vi "AddLifetimeData.vi"(0 "lower time (ms)":dbl, 1 "upper time (ms)":dbl, 2 "Decay":u32[][](array[numeric]), 3 "RAW data":T1) -> (8 "Decay out":u32[][](array[numeric]))   [LabVIEW 2009]
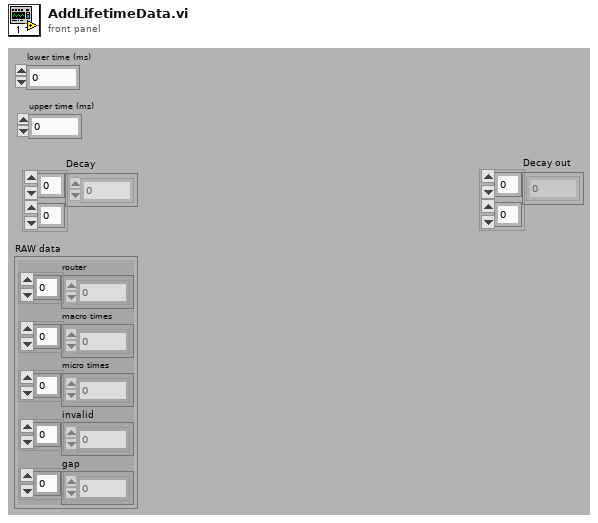
[diagram p1: front panel]
types:
  T1 = cluster{"router":u8[], "macro times":dbl[], "micro times":u16[], "invalid":dbl[], "gap":dbl[]}
  T2 = typedef "Settings.ctl" = cluster{"threshold":cluster{"max":u32, "min":u32}, "RGB or false color":bool, "16bit":bool, "log/lin axis":u16, "spotsize button":bool, "Pixelsize":u16, "autoscale x":bool, "autoscale y":bool, "correlation":bool, "ADC-Resolution":i32, "F2-lifetime":cluster{"display tau":bool, "display F2":bool, "Palette Number lifetime":enum32{"Gray", "Binary", "Gradient", "Rainbow", "Temperature"}, "Palette Number F2":enum32{"Gray", "Binary", "Gradient", "Rainbow", "Temperature"}, "max tau-Value":dbl, "min tau-Value":dbl, "max F2-Value":dbl, "min F2-Value":dbl}, "TAC-Window 1":u16, "TAC-Window 2":u16, "false color palette":cluster{"1":u32, "2":u32, "3":u32, "4":u32, "5":u32, "6":u32, "7":u32, "8":u32, "8 2":u32, "8 3":u32, "8 4":u32, "8 5":u32}, "rebinning":dbl}
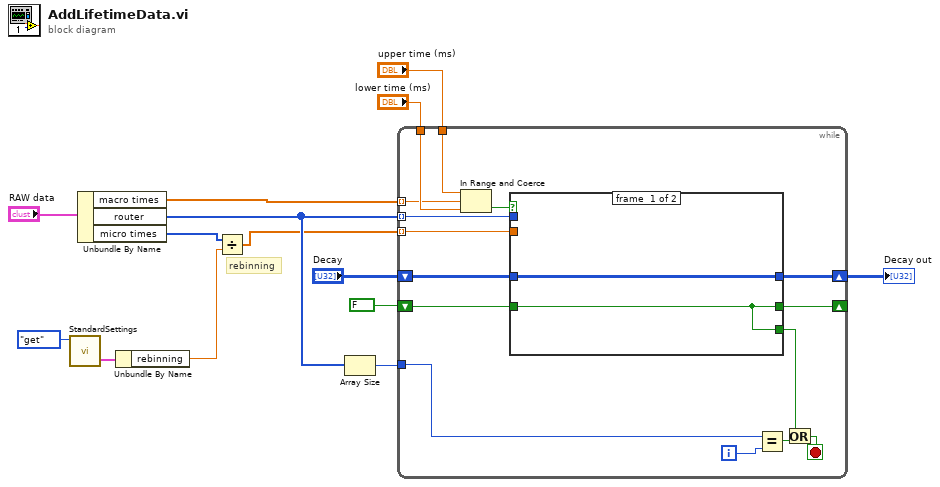
[diagram p0: block diagram]
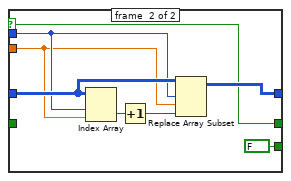
[diagram p2: hidden frame]
diagram:
  # "rebinning"
  n1 = call "StandardSettings.vi"("Enum"=enum16{"Load", "get", "Save", "set"}."get") -> ("StandardSettings"=w3:T2)  [unwired: 4 in]
  n2 = Unbundle By Name("RAW data") -> ("macro times"=w11:dbl[], "router"=w7:u8[], "micro times"=w5:u16[])
  n3 = Unbundle By Name(w3) -> ("rebinning"=w1:dbl)
  n4 = Divide(x=w5, y=w1) -> (x/y=w4:dbl[])
  n5 = Array Size(array=w7) -> (size(s)=w8:i32)
  n6 = while {
    tunnel: "lower time (ms)" -> [w29]
    tunnel: "upper time (ms)" -> [w15]
    shift-right: [w23] -> w6
    shift-left: "Decay" -> [w24]
    tunnel: w11 -> [w25] mode=indexing
    tunnel: w7 -> [w27] mode=indexing
    tunnel: w4 -> [w26] mode=indexing
    shift-right: [w22] -> _
    shift-left: FALSE -> [w21]
    tunnel: w8 -> [w20]
    i -> [w19]
    stop <- w18 stop-if-true
    n7 = In Range and Coerce(upper limit=w15, x=w25, lower limit=w29) -> (In Range?=w28:bool)  [unwired: 1 out]
    n8 = case shown="True" w28 {
      selector: w28 -> [_ w34]
      tunnel: w27 -> [_ w36]
      tunnel: w26 -> [_ w32]
      tunnel: w24 -> [w31 w38]
      tunnel: [w31 w35] -> w23
      tunnel: [w30 w34] -> w22
      tunnel: w21 -> [w30 _]
      tunnel: [w30 FALSE] -> w17
      frame #0 {
      }
      frame #1 {
        n9 = Index Array(array=w38, index (row)=w36, index (col)=w32) -> (element=w39:u32)
        n10 = Increment(x=w39) -> (x+1=w37:u32)
        n11 = Replace Array Subset(array=w38, new element=w37, index (row)=w36, index (col)=w32) -> (w35:u32[][])
      }
    }
    n12 = Equal?(x=w20, y=w19) -> (x = y?=w16:bool)
    n13 = Or(x=w17, y=w16) -> (x .or. y?=w18:bool)
  }
  "Decay out" <- w6
